vi "sub_CloseDevices.vi"(8 "error in (no error)":errorcluster, 10 "Dynamic data":T1, 11 "Input parameters":T2={"Measurement type"=enum."Test", "Sensor type"=enum."HPK_8in_256", "Identifier"="test.txt", "Open after execution?"=FALSE, "Plot after execution?"=FALSE, "Display channel"=0, "Voltage Delay (s)"=0.5, "Switch Delay (s)"=0.01, "VISA resource name source"="", "VISA resource name DMM"="", "VISA resource name LCR"="", "Compliance  Level (uA)"=10.0, "Voltage Limit (V)"=1000.0, "Data storage location"="", "Scan voltages"="", "Use source as DMM?"=FALSE, "Single channel?"=FALSE, "LCR signal frequenzy (Hz)"=10.0, "DMM device"=enum."Keithley2001"} {"Voltage Limit (V)" format="%#_13g"; "Voltage Delay (s)" format="%#_13g"; "Switch Delay (s)" format="%#_13g"}) -> (0 "error out":errorcluster, 2 "Dynamic data":T1, 3 "Input parameters":T2={"Measurement type"=enum."Test", "Sensor type"=enum."HPK_8in_256", "Identifier"="test.txt", "Open after execution?"=FALSE, "Plot after execution?"=FALSE, "Display channel"=0, "Voltage Delay (s)"=0.5, "Switch Delay (s)"=0.01, "VISA resource name source"="", "VISA resource name DMM"="", "VISA resource name LCR"="", "Compliance  Level (uA)"=10.0, "Voltage Limit (V)"=1000.0, "Data storage location"="", "Scan voltages"="", "Use source as DMM?"=FALSE, "Single channel?"=FALSE, "LCR signal frequenzy (Hz)"=10.0, "DMM device"=enum."Keithley2001"} {"Voltage Limit (V)" format="%#_13g"; "Voltage Delay (s)" format="%#_13g"; "Switch Delay (s)" format="%#_13g"})   [LabVIEW 2016]
uses:
  Input_parameters.ctl
  Dynamic_data.ctl
  <instrlib>/Keithley 24XX/Keithley 24XX.lvlib
  instr.lib/Agilent E4980/Agilent E4980.lvlib
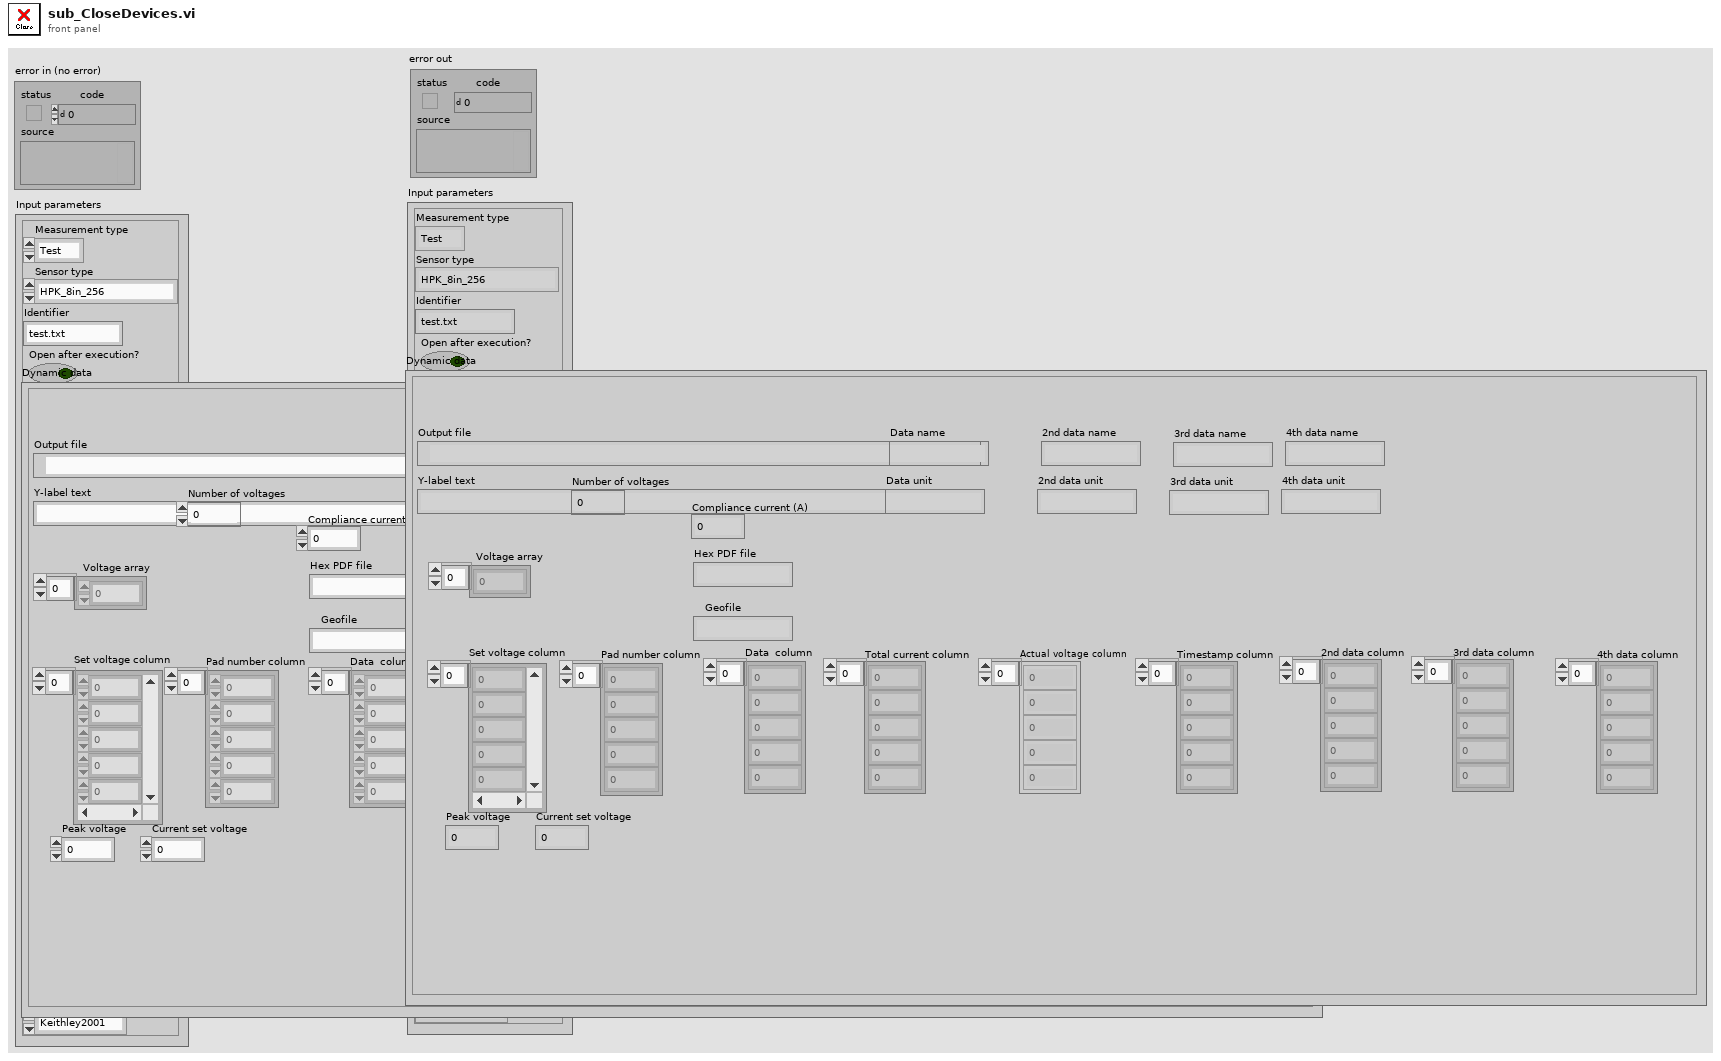
[diagram p1: front panel]
types:
  T1 = typedef "Dynamic_data.ctl" = cluster{"Output file":path, "Y-label text":string, "Current set voltage":dbl, "Set voltage column":dbl[], "Pad number column":dbl[], "Data  column":dbl[], "Number of voltages":i32, "Compliance current (A)":dbl, "Geofile":string, "Peak voltage":dbl, "Hex PDF file":string, "Voltage array":dbl[], "Total current column":dbl[], "Timestamp column":dbl[], "Data name":string, "Data unit":string, "2nd data column":dbl[], "2nd data name":string, "2nd data unit":string, "3rd data column":dbl[], "4th data column":dbl[], "3rd data name":string, "3rd data unit":string, "4th data name":string, "4th data unit":string, "Actual voltage column":dbl[]}
  T2 = typedef "Input_parameters.ctl" = cluster{"Measurement type":enum16{"IV", "CV", "Test"}, "Sensor type":enum16{"HPK_6in_135", "HPK_8in_256", "INF_8in_256", "Diode"}, "Identifier":string, "Open after execution?":bool, "Plot after execution?":bool, "Display channel":i32, "Voltage Delay (s)":dbl, "Switch Delay (s)":dbl, "VISA resource name source":refnum<visa-resource-name>, "VISA resource name DMM":refnum<visa-resource-name>, "VISA resource name LCR":refnum<visa-resource-name>, "Compliance  Level (uA)":dbl, "Voltage Limit (V)":dbl, "Data storage location":string, "Scan voltages":string, "Use source as DMM?":bool, "Single channel?":bool, "LCR signal frequenzy (Hz)":dbl, "DMM device":enum16{"Keithley2001", "Keithley2450", "Keithley2410"}}
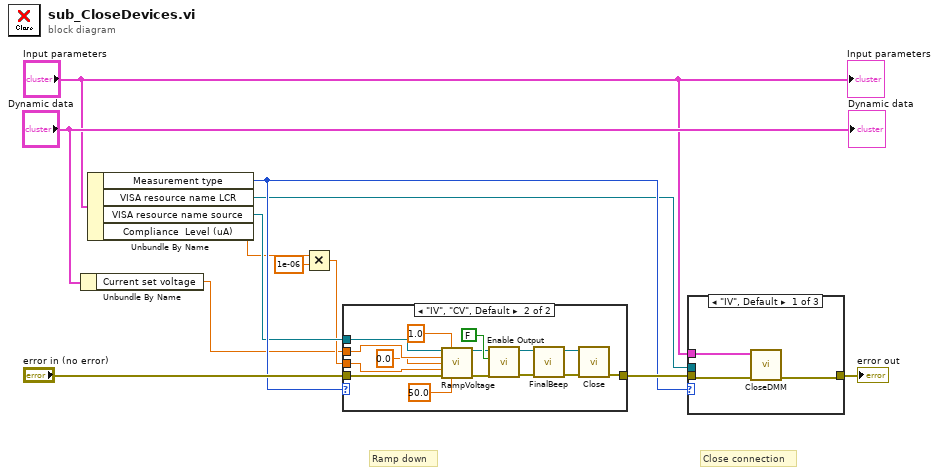
[diagram p0: block diagram]
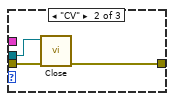
[diagram p3: hidden frame]
diagram:
  # "Close connection"
  # "Ramp down"
  n1 = Unbundle By Name("Dynamic data") -> ("Current set voltage"=w3:dbl)
  n2 = Unbundle By Name("Input parameters") -> ("Measurement type"=w9:enum16{"IV", "CV", "Test"}, "VISA resource name LCR"=w1:refnum<visa-resource-name>, "VISA resource name source"=w8:refnum<visa-resource-name>, "Compliance  Level (uA)"=w6:dbl)
  n3 = Multiply(x=w6, y=1e-06) -> (x*y=w5:dbl)
  n4 = case shown="\"IV\", \"CV\", Default" w9 {
    tunnel: w8 -> [_ w27]
    tunnel: "error in (no error)" -> [w13 w28]
    tunnel: [w13 w18] -> w12
    tunnel: w5 -> [_ w25]
    tunnel: w3 -> [_ w26]
    frame "Test" {
    }
    frame "IV", "CV", Default {
      n5 = call "RampVoltage.vi"("VISA resource name"=w27, "Delay (s)"=1.0, "Current voltage (V)"=w26, "Target voltage (V)"=0.0, "Compliance Current (A)"=w25, "error in (no error)"=w28, "Step size (V)"=50.0) -> ("VISA resource name out"=w19:refnum<visa-resource-name>, "error out"=w20:errorcluster)  [unwired: 6 in, 1 out]
      n6 = call <instrlib>:"Enable Output.vi"("error in (no error)"=w20, "Enable Output (T: Enable)"=FALSE ("Enable Output"), "VISA resource name"=w19) -> ("error out"=w17:errorcluster, "VISA resource name out"=w16:refnum<visa-resource-name>)  [unwired: 7 in]
      n7 = call "FinalBeep.vi"("error in (no error)"=w17, "VISA resource name"=w16) -> ("error out"=w14:errorcluster, "VISA resource name out"=w15:refnum<visa-resource-name>)  [unwired: 8 in]
      n8 = call <instrlib>:"Close.vi"("error in (no error)"=w14, "VISA resource name"=w15) -> ("error out"=w18:errorcluster)  [unwired: 9 in]
    }
  }
  n9 = case shown="\"IV\", Default" w9 {
    tunnel: w12 -> [w30 w34 w35]
    tunnel: [w31 w33 w35] -> w10
    tunnel: "Input parameters" -> [w29 _ _]
    tunnel: w1 -> [_ w32 _]
    frame "IV", Default {
      n10 = call "CloseDMM.vi"("error in (no error)"=w30, "Input parameters"=w29) -> ("error out"=w31:errorcluster)  [unwired: 9 in]
    }
    frame "CV" {
      n11 = call <instrlib>:"Close.vi"("error in (no error)"=w34, "VISA resource name"=w32) -> ("error out"=w33:errorcluster)  [unwired: 9 in]
    }
    frame "Test" {
    }
  }
  "error out" <- w10
  "Input parameters" <- "Input parameters"
  "Dynamic data" <- "Dynamic data"
